vi "SRV_Read Sensors Config File.vi"(0 "Sensors Config File Path":path, 11 "error in (no error)":errorcluster={"status"=TRUE, "code"=42, "source"="LPD_String to Enum.vi\r\nCall Chain:\r\nSRV_Sensor Config GUI.vi >> SRV_Sensor Name to Sensor Name Enum.vi >> LPD_String to Enum.vi\r\n\r\nThe value \"\" is not valid for \"Sensor to Edit\"."}) -> (4 "Sensors Config File Path out":path, 8 "Sensors Config":T1[](array[typedef]) {"Register" format="%.0x"; "I2C Address" format="%.0x"; "Sample Period (ms)" min=10 max=60000 step=1; "Digital Mask" format="%.0x"; "Channel" format="%.0x"}, 10 "Cancelled?":bool, 15 "error out":errorcluster={"status"=TRUE, "code"=42, "source"="LPD_String to Enum.vi\r\nCall Chain:\r\nSRV_Sensor Config GUI.vi >> SRV_Sensor Name to Sensor Name Enum.vi >> LPD_String to Enum.vi\r\n\r\nThe value \"\" is not valid for \"Sensor to Edit\"."})   [LabVIEW 2014]
uses:
  SRV_Sensor Config Cluster.ctl
  SRV_Sensor Analog-Digital.ctl
  SRV_Sensor Sampling Mode.ctl
  SRV_Sensor View Config Cluster.ctl
  SRV_Sensors Names.ctl
  SRV_Sensor PicoC Shared Var Type.ctl
  SRV_Sensor Number of Bytes.ctl
  SRV_Sensor Integer Word Type.ctl
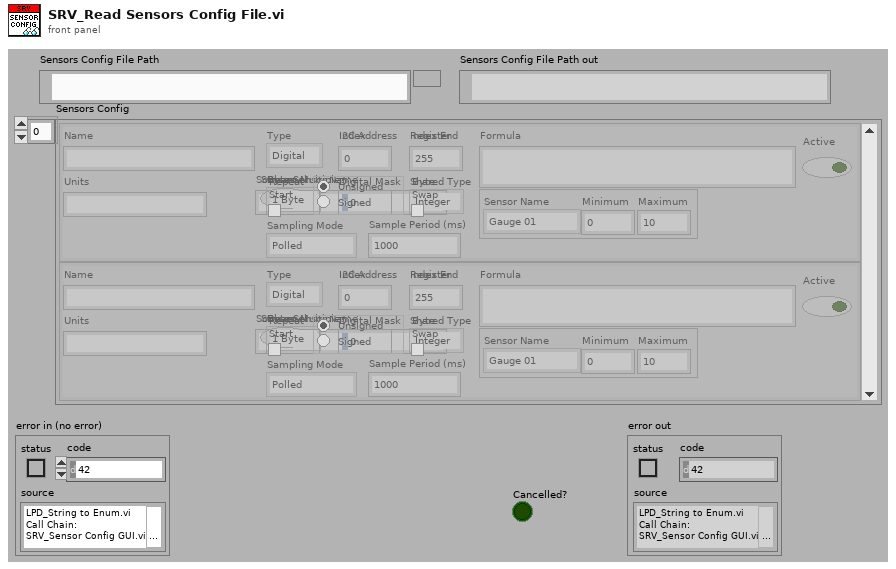
[diagram p1: front panel]
types:
  T1 = typedef "SRV_Sensor Config Cluster.ctl" = cluster{"Name":string, "A/D":T2, "I2C Address":u8, "Register":u8, "Channel":u8, "Digital Mask":u16, "Units":string, "Sampling Mode":T3, "Sample Period (ms)":u32, "Formula":string, "Sensor View Config":T4, "Active":bool, "PicoC Shared Var Type":T6, "Index":u8, "Stream Multiple?":bool, "Index End":u8, "Bytes":T7, "Source Sensor Name":string, "Repeat Start":bool, "Integer Word Type":T8, "Byte Swap":bool}
  T2 = typedef "SRV_Sensor Analog-Digital.ctl" = enum16{"Digital", "Analog", "PicoC Shared", "Calculated"}
  T3 = typedef "SRV_Sensor Sampling Mode.ctl" = enum16{"Polled", "Streaming"}
  T4 = typedef "SRV_Sensor View Config Cluster.ctl" = cluster{"Sensor Name":T5, "Minimum":dbl, "Maximum":dbl}
  T5 = typedef "SRV_Sensors Names.ctl" = enum16{"Gauge 01", "Gauge 02", "Gauge 03", "Gauge 04", "Meter 01", "Meter 02", "Meter 03", "Meter 04", "Numeric 01", "Numeric 02", "Numeric 03", "Numeric 04", "Numeric 05", "Numeric 06", "Numeric 07", "Numeric 08", "Boolean 01", "Boolean 02", "Boolean 03", "Boolean 04", "Boolean 05", "Boolean 06", "Boolean 07", "Boolean 08", "Boolean 09", "Boolean 10", "Boolean 11", "Boolean 12", "Boolean 13", "Boolean 14", "Boolean 15", "Boolean 16", "Boolean 17", "Boolean 18", "Boolean 19", "Boolean 20", "Boolean 21", "Boolean 22", "Boolean 23", "Boolean 24", "Boolean 25", "Boolean 26", "Boolean 27", "Boolean 28", "Boolean 29", "Boolean 30", "Boolean 31", "Boolean 32"}
  T6 = typedef "SRV_Sensor PicoC Shared Var Type.ctl" = enum16{"String", "Integer", "Float"}
  T7 = typedef "SRV_Sensor Number of Bytes.ctl" = enum16{"1 Byte", "2 Bytes"}
  T8 = typedef "SRV_Sensor Integer Word Type.ctl" = enum32{"Unsigned", "Signed"}
  T9 = enum16{"open", "open or create", "create or replace", "create", "open (read only)"}
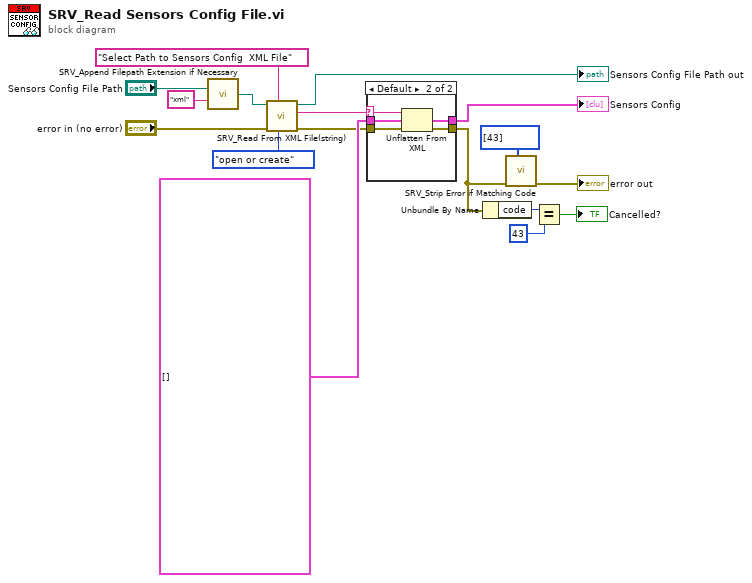
[diagram p0: block diagram]
diagram:
  n1 = call "SRV_Append Filepath Extension if Necessary.vi"("Filepath"="Sensors Config File Path", "Extension"="xml") -> ("Filepath with Extension"=w7:path)  [unwired: 13 in]
  n2 = call "SRV_Read From XML File(string).vi"("function (open-read-only:4)"=T9."open or create", "Prompt"="Select Path to Sensors Config  XML File", "error in (no error)"="error in (no error)", "XML File Path"=w7) -> ("error out"=w9:errorcluster, "XML Elements"=w5:string, "XML File Path(duplicate)"=→"Sensors Config File Path out":path)  [unwired: 5 in]
  n3 = case shown="Default" w5 {
    selector: w5 -> [_ w20]
    tunnel: T1[] [] ("Sensors Config 2") -> [w18 w24]
    tunnel: [w18 w23] -> w14
    tunnel: [w19 w22] -> w2
    tunnel: w9 -> [w19 w21]
    frame "" {
    }
    frame Default {
      n4 = Unflatten From XML(xml string=w20, type=w24, error in (no error)=w21) -> (value=w23:T1[], error out=w22:errorcluster)
    }
  }
  "Sensors Config" <- w14
  n5 = Unbundle By Name(w2) -> ("code"=w13:i32)
  n6 = call "SRV_Strip Error if Matching Code.vi"("error in (no error)"=w2, "Strip Codes"=i32[] [43]) -> ("error out"=→"error out":errorcluster)  [unwired: 8 in]
  n7 = Equal?(x=w13, y=43) -> (x = y?=→"Cancelled?":bool)
